vi "Hall of Bar sample Test.vi"(8 "error in (no error)":errorcluster) -> (0 "error out":errorcluster)   [LabVIEW 2016, in "Hall Effect Library.lvlib"]
uses:
  Hall Effect Library.lvlib
  Controls/Measurement.ctl
  Public/Controls/Data Items.ctl
  Public/Controls/Tests.ctl
  Global Variables/Test Settings.vi
  Global Variables/Hall Effect Data.vi
  Global Variables/Instrument Locations.vi
panel:
  out "Test Step":T1(ring)
  out "Measurement":T2
  out "Soak Until":timestamp
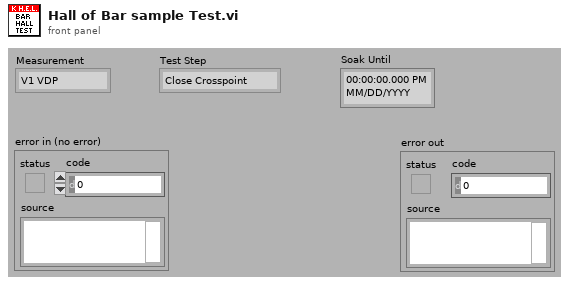
[diagram p1: front panel]
types:
  T1 = enum16{"Close Crosspoint", "Soak 1", "Zero Ammeter", "Zero Voltmeter", "I-SRC On", "Adjust potentiometer to 0V ", "Init Ammeter", "Soak 2", "Measure I", "Measure V", "I-SRC Off", "Open Crosspoint", "Done"}
  T2 = typedef "Hall Effect Library.lvlib/Measurement.ctl" = enum16{"V1 VDP", "V2 VDP", "V3 VDP", "V4 VDP", "V5 VDP", "V6 VDP", "V7 VDP", "V8 VDP", "V1 HE", "V2 HE", "V3 HE", "V4 HE", "V5 HE", "V6 HE", "V7 HE", "V8 HE", "V1 Res Bar", "V1 Hall Bar", "V1 Res 6-Cot", "V2 Res 6-Cot", "V3 Res 6-Cot", "V4 Res 6-Cot", "V1 Hall 6-Cot", "V2 Hall 6-Cot", "V3 Hall 6-Cot", "V4 Hall 6-Cot", "V5 Hall 6-Cot", "V6 Hall 6-Cot", "V7 Hall 6-Cot", "V8 Hall 6-Cot", "V1 Res 8-Cot", "V2 Res 8-Cot", "V3 Res 8-Cot", "V4 Res 8-Cot", "V1 Hall 8-Cot", "V2 Hall 8-Cot", "V3 Hall 8-Cot", "V4 Hall 8-Cot"}
  T3 = typedef "Hall Effect Library.lvlib/Resisitivity.ctl" = enum16{"Low", "High"}
  T4 = enum16{"Close Crosspoint", "Soak 1", "Zero Ammeter", "Zero Voltmeter", "I-SRC On", "Init Ammeter", "Soak 2", "Measure I", "Measure V", "I-SRC Off", "Open Crosspoint", "Done"}
  T5 = typedef "Hall Effect Library.lvlib/Tests.ctl" = enum16{"Van Der Pauw", "Hall Effect", "Bar Sample Resistivity", "Bar Sample Hall ", "6-Contact Sample Resistivity", "6-Contact Sample Hall", "8-Contact Sample Resistivity", "8-Contact Sample Hall", ""}
  T6 = typedef "Hall Effect Library.lvlib/Data Items.ctl" = enum16{"V1 Van Der Pauw", "V2 Van Der Pauw", "V3 Van Der Pauw", "V4 Van Der Pauw", "V5 Van Der Pauw", "V6 Van Der Pauw", "V7 Van Der Pauw", "V8 Van Der Pauw", "V1 Hall Effect", "V2 Hall Effect", "V3 Hall Effect", "V4 Hall Effect", "V5 Hall Effect", "V6  Hall Effect", "V7 Hall Effect", "V8 Hall Effect", "V1 Res Bar", "V1 Hall Bar", "V1 Res 6-Cot", "V2 Res 6-Cot", "V3 Res 6-Cot", "V4 Res 6-Cot", "V1 Hall 6-Cot", "V2 Hall 6-Cot", "V3 Hall 6-Cot", "V4 Hall 6-Cot", "V5 Hall 6-Cot", "V6 Hall 6-Cot", "V7 Hall 6-Cot", "V8 Hall 6-Cot", "V1 Res 8-Cot", "V2 Res 8-Cot", "V3 Res 8-Cot", "V4 Res 8-Cot", "V1 Hall 8-Cot", "V2 Hall 8-Cot", "V3 Hall 8-Cot", "V4 Hall 8-Cot", "Van Der Pauw Results", "Hall Effect Results", "Bar Sample Resistivity Results", "Bar Sample Hall Results", "6-Contact Resistivity Results", "6-Contact Hall Results", "8-Contact Resistivity Results", "8-Contact Hall Results"}
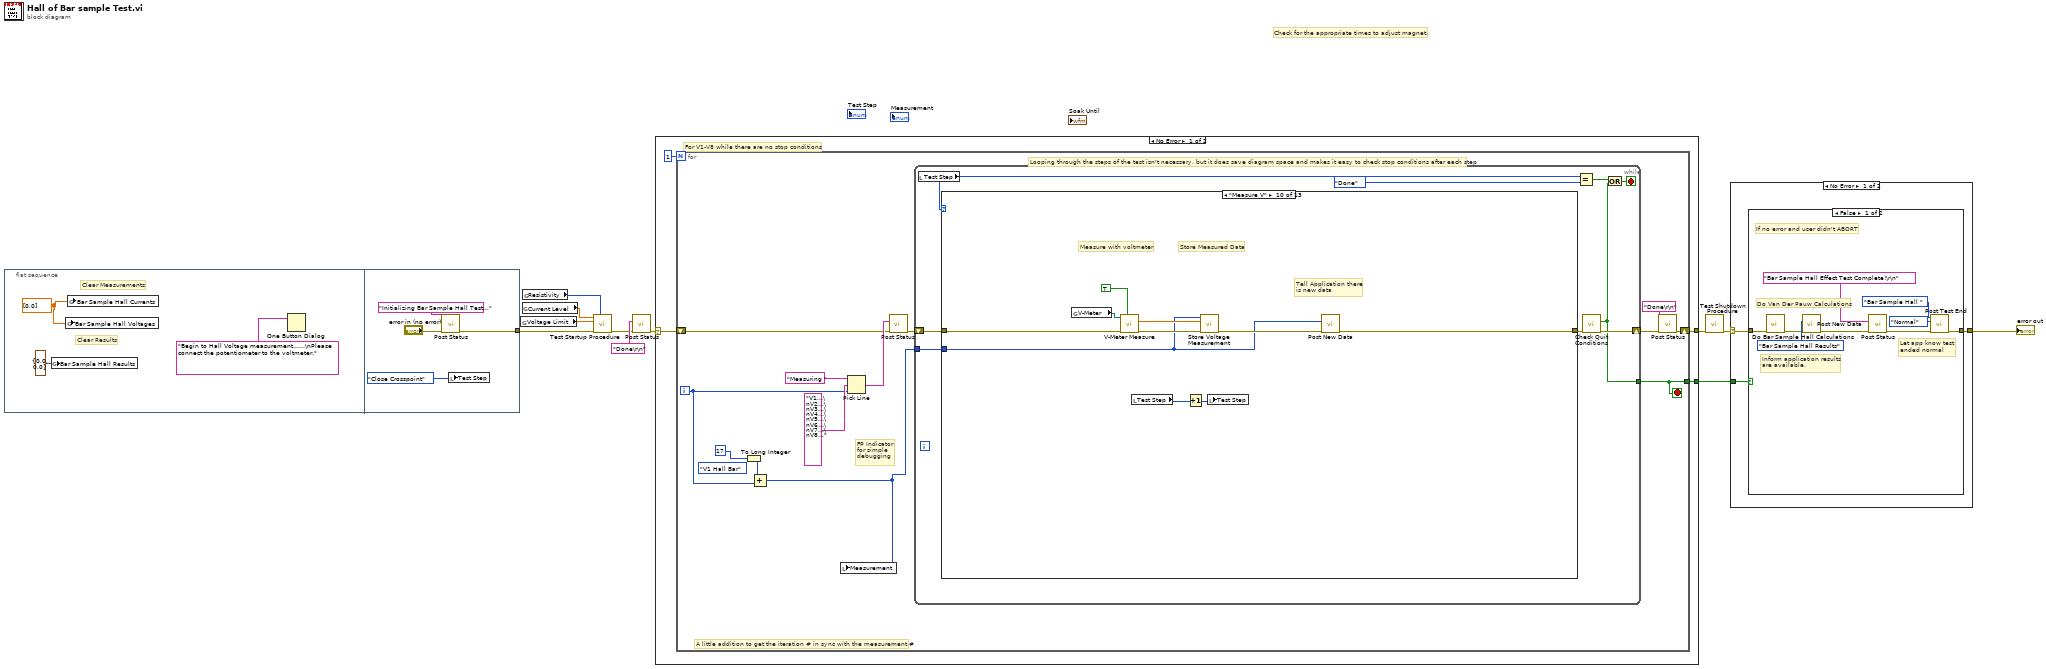
[diagram p0: block diagram]
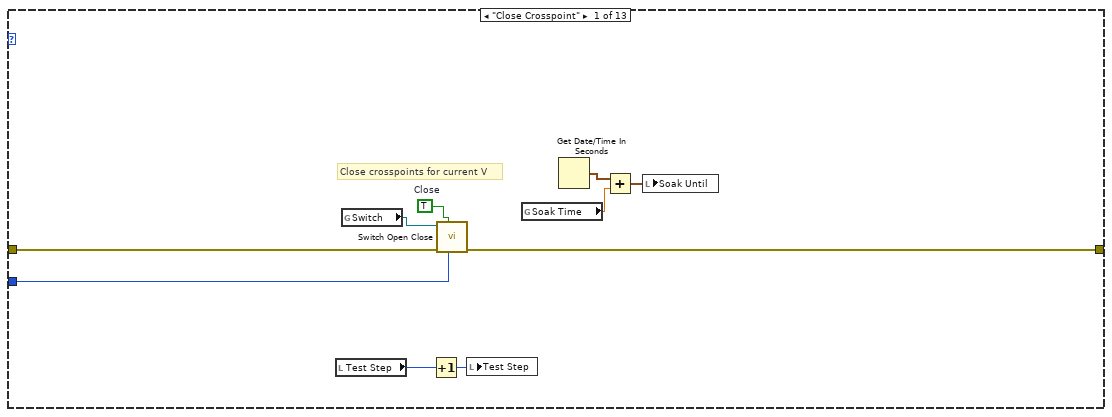
[diagram p2: hidden frame]
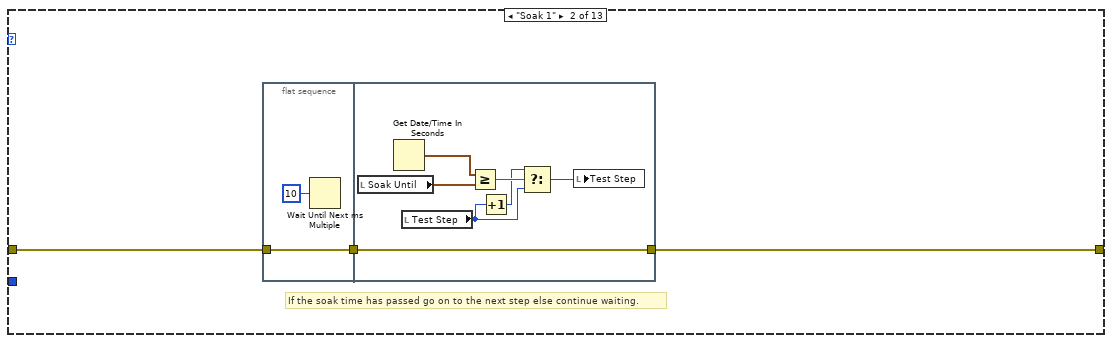
[diagram p3: hidden frame]
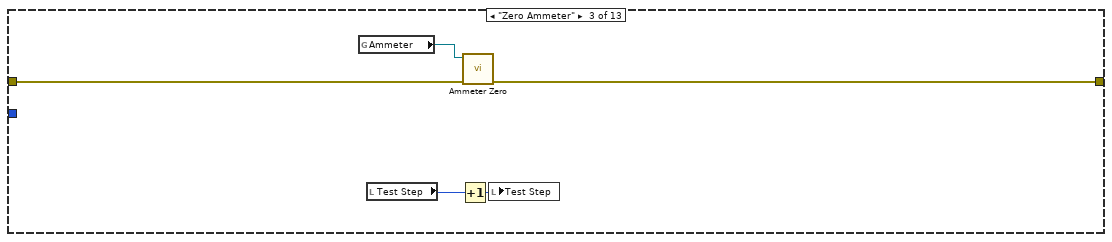
[diagram p4: hidden frame]
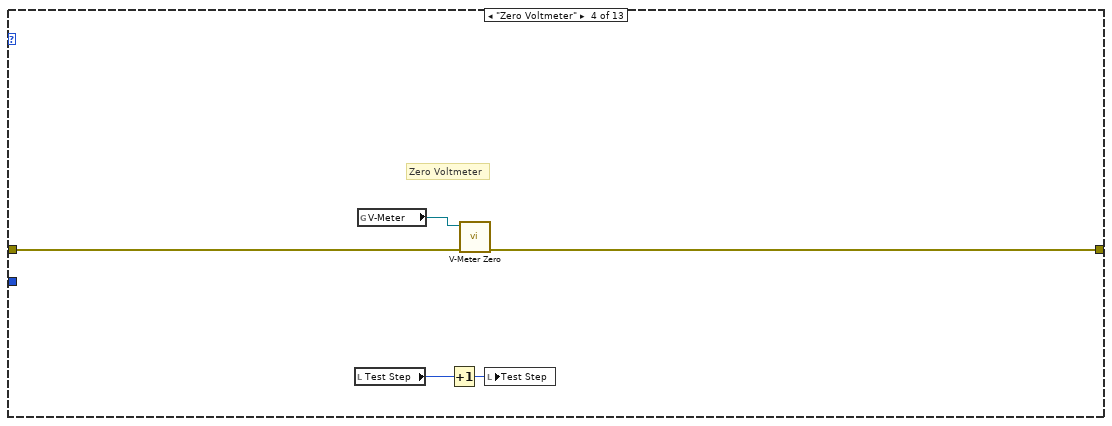
[diagram p5: hidden frame]
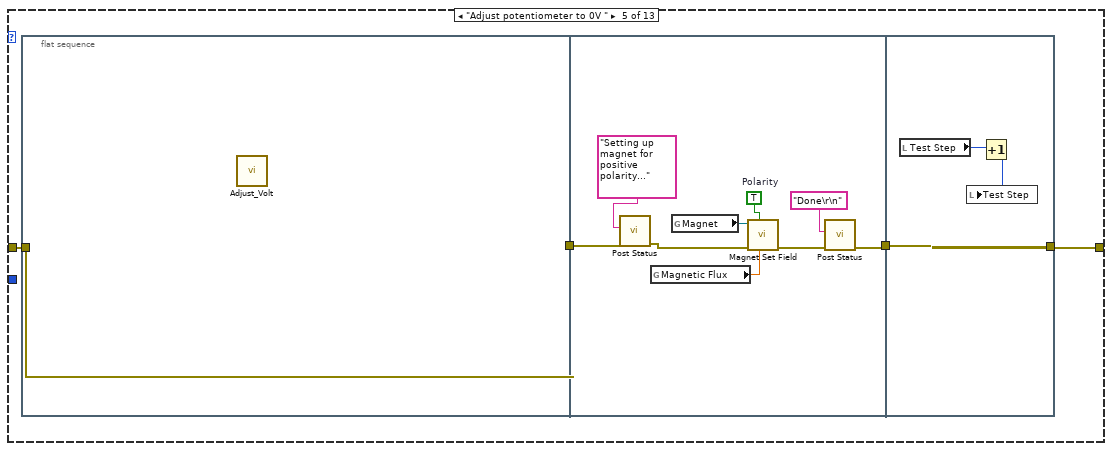
[diagram p6: hidden frame]
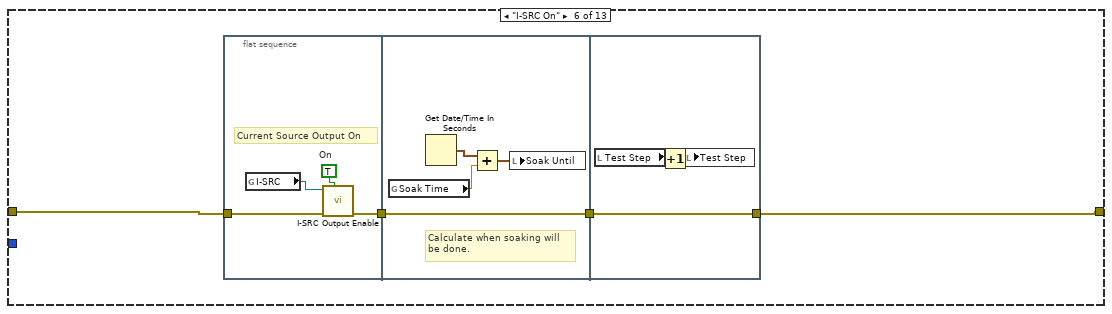
[diagram p7: hidden frame]
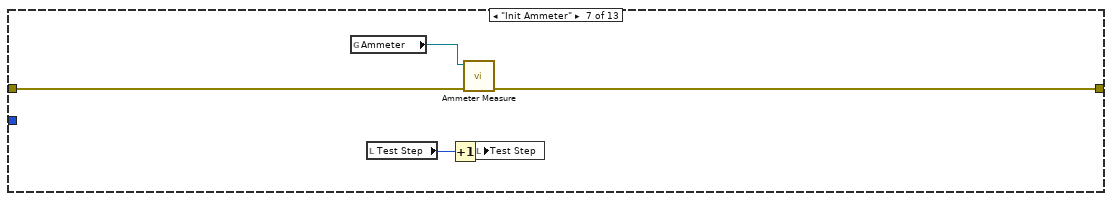
[diagram p8: hidden frame]
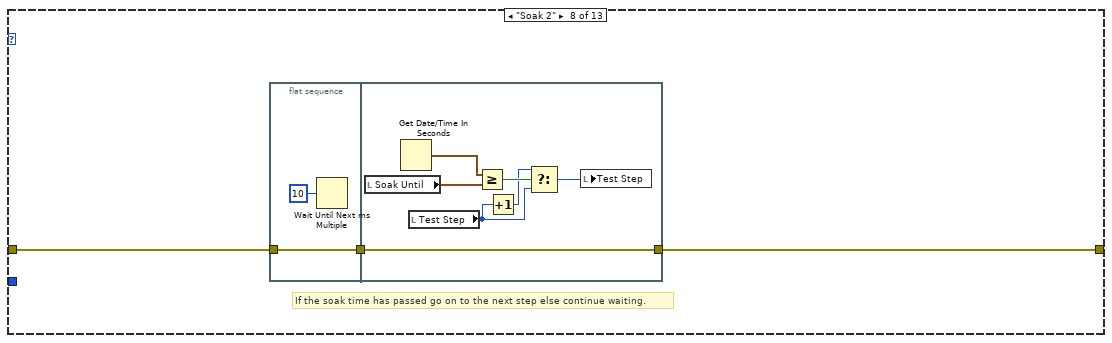
[diagram p9: hidden frame]
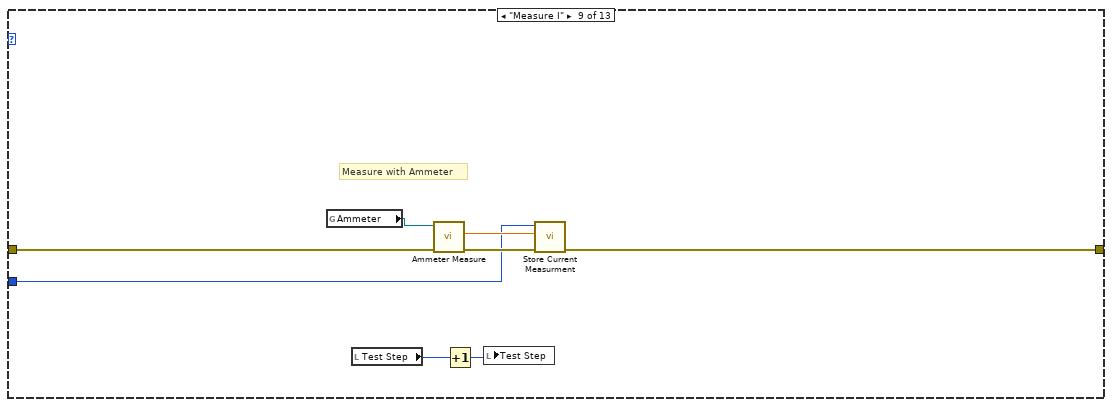
[diagram p10: hidden frame]
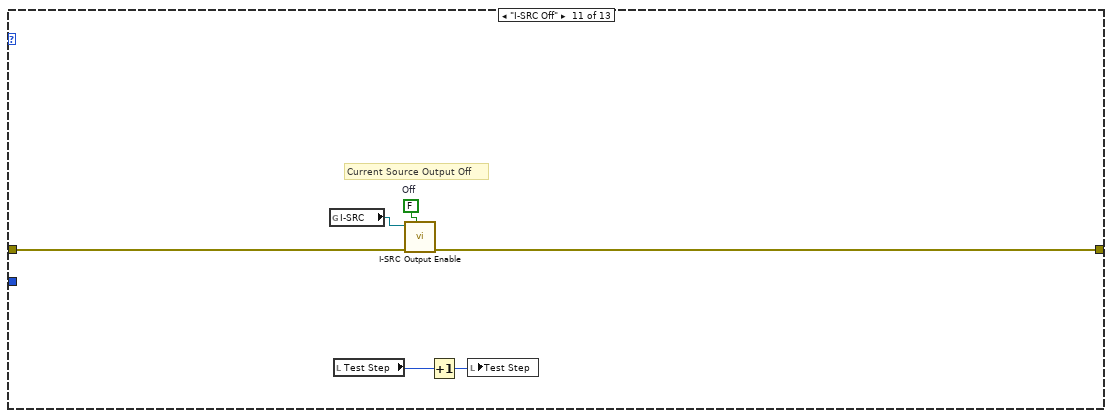
[diagram p11: hidden frame]
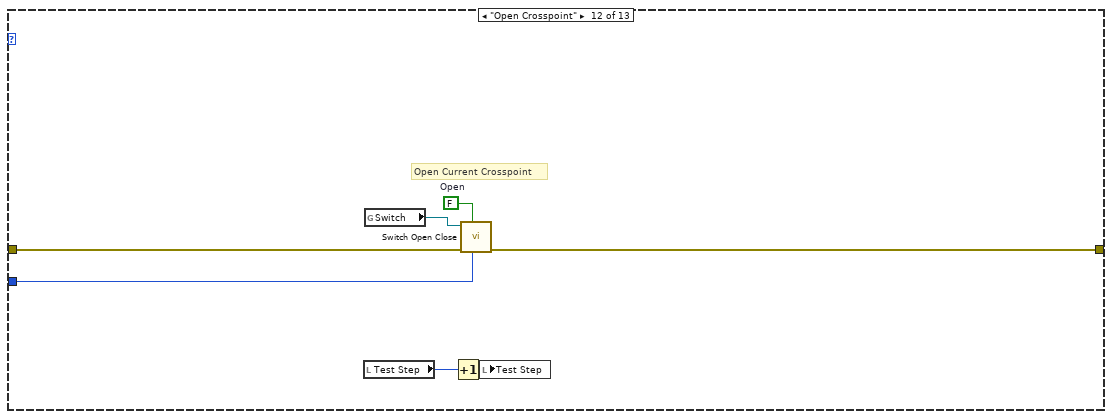
[diagram p12: hidden frame]
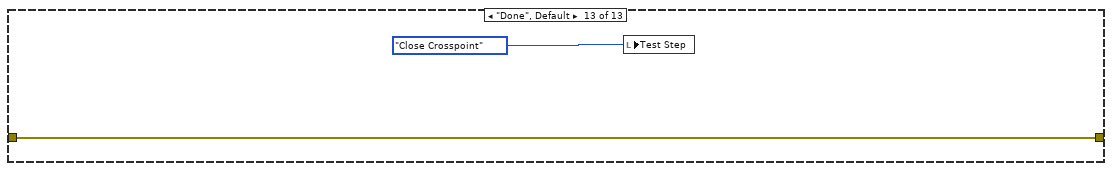
[diagram p13: hidden frame]
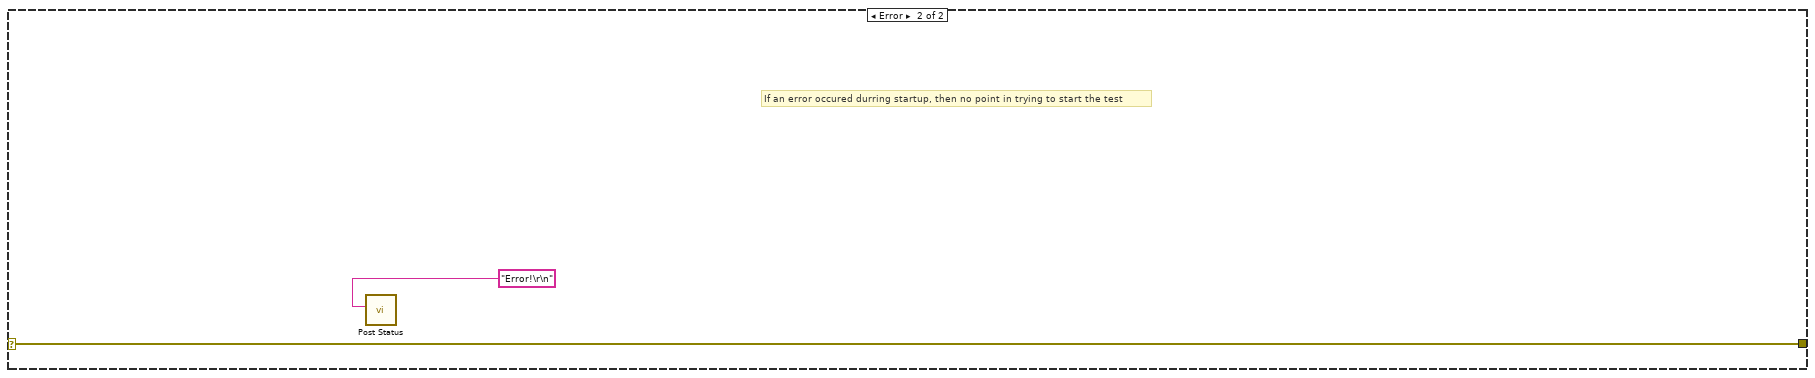
[diagram p14: hidden frame]
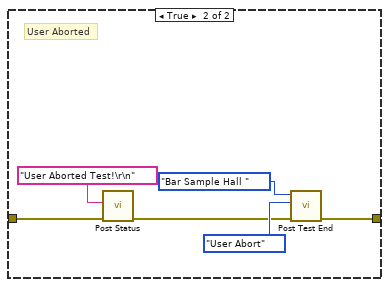
[diagram p15: hidden frame]
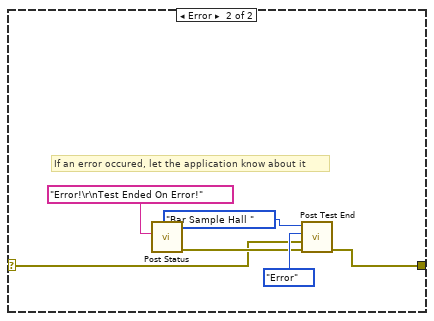
[diagram p16: hidden frame]
diagram:
  # "Check for the appropriate times to adjust magnet."
  n1 = flat-sequence {
    tunnel: [w18] -> w5
    frame #0 {
      w14 = dbl[] [0.0] ("Bar Sample Hall Currents")
      # "Clear Results"
      # "Clear Measurements"
      n2 = global write "Hall Effect Data.vi" "Bar Sample Hall Results"(cluster{"n/p":dbl, "uH":dbl} {"n/p"=0.0, "uH"=0.0} ("Bar Sample Hall Results")) -> ()
      n3 = global write "Hall Effect Data.vi" "Bar Sample Hall Voltages"(w14) -> ()
      n4 = global write "Hall Effect Data.vi" "Bar Sample Hall Currents"(w14) -> ()
      n5 = One Button Dialog(message="Begin to Hall Voltage measurement......\nPlease connect the potentiometer to the voltmeter.") -> ()  [unwired: 1 in, 1 out]
    }
    frame #1 {
      n6 = call "Post Status.vi"("error in (no error)"="error in (no error)", "Status Message"="Initializing Bar Sample Hall Test...") -> ("error out"=w18:errorcluster)  [unwired: 9 out]
      n7 = local write "Test Step"(T1."Close Crosspoint" ("Test Step")) -> ()
    }
  }
  n8 = global read "Test Settings.vi" "Voltage Limit"() -> (w6:dbl)
  n9 = global read "Test Settings.vi" "Current Level"() -> (w7:dbl)
  n10 = global read "Test Settings.vi" "Resistivity"() -> (w8:T3)
  n11 = call "Test Startup Procedure.vi"("Resistivity"=w8, "error in (no error)"=w5, "Voltage Limit"=w6, "Current Level"=w7) -> ("error out"=w3:errorcluster)  [unwired: 7 out]
  n12 = call "Post Status.vi"("error in (no error)"=w3, "Status Message"="Done\r\n") -> ("error out"=w9:errorcluster)  [unwired: 9 out]
  n13 = case shown="No Error" w9 {
    selector: w9 -> [w20 w160]
    tunnel: [w22 w160] -> w2
    tunnel: [w21 _] -> w10
    frame No Error {
      # "For V1-V8 while there are no stop conditions"
      n14 = for {
        N: 1 -> [_]
        shift-right: [w28] -> w22
        shift-left: w20 -> [w24]
        tunnel: [w25] -> w21
        i -> [w30]
        stop <- w25 stop-if-true
        (unwired) Measurement."V1 Hall Bar" ("Measurement")
        # "A little addition to get the iteration # in sync with the measurement #"
        # "FP Indicator\nfor simple\ndebugging"
        # "Looping through the steps of the test isn't necessary, but it does save diagram space and makes it easy to check stop conditions after each step"
        n15 = To Long Integer(number=17) -> (32bit integer=w31:i32)
        n16 = Add(x=w31, y=w30) -> (x+y=w26:i32)
        n17 = local write "Measurement"(w26) -> ()
        n18 = Pick Line(string ("")="Measuring ", multi-line string="V1...\nV2...\nV3...\nV4...\nV5...\nV6...\nV7...\nV8...", line index=w30) -> (output string=w33:string)
        n19 = call "Post Status.vi"("error in (no error)"=w24, "Status Message"=w33) -> ("error out"=w32:errorcluster)  [unwired: 9 out]
        n20 = while {
          shift-right: [w42] -> w27
          shift-left: w32 -> [w44]
          tunnel: w26 -> [w43]
          tunnel: [w38] -> w25
          stop <- w41 stop-if-true
          n21 = local read "Test Step"() -> (w39:T1)
          n22 = case shown="\"Measure V\"" w39 {
            tunnel: [w52 w55 w70 w74 w79 w96 w112 w115 w130 w138 w146 w154 w158] -> w37
            tunnel: w44 -> [w51 w56 w71 w75 w80 w97 w113 w116 w132 w142 w147 w153 w158]
            tunnel: w43 -> [w50 _ _ _ _ _ _ _ w128 w137 _ w152 _]
            frame "Close Crosspoint" {
              w53 = TRUE  # Close
              # "Close crosspoints for current V"
              n23 = local read "Test Step"() -> (w48:T1)
              n24 = global read "Instrument Locations.vi" "Switch"() -> (w54:refnum<visa-resource-name>)
              n25 = Increment(x=w48) -> (x+1=w49:T1)
              n26 = call "Switch Open Close.vi"("Measurement"=w50, "Open/Close (F: Open)"=w53, "error in (no error)"=w51, "VISA resource name in"=w54) -> ("error out"=w52:errorcluster)  [unwired: 7 out]
              n27 = local write "Test Step"(w49) -> ()
              n28 = global read "Test Settings.vi" "Soak Time"() -> (w46:dbl)
              n29 = Get Date/Time In Seconds() -> (seconds since 1Jan1904=w45:timestamp)
              n30 = Add(x=w45, y=w46) -> (x+y=w47:timestamp)
              n31 = local write "Soak Until"(w47) -> ()
            }
            frame "Soak 1" {
              # "If the soak time has passed go on to the next step else continue waiting."
              n32 = flat-sequence {
                tunnel: w56 -> [w58]
                tunnel: [w58] -> w57
                tunnel: [w62] -> w55
                tunnel: w57 -> [w62]
                frame #0 {
                  n33 = Wait Until Next ms Multiple(millisecond multiple=u32 10) -> ()  [unwired: 1 out]
                }
                frame #1 {
                  n34 = local read "Soak Until"() -> (w65:timestamp)
                  n35 = Get Date/Time In Seconds() -> (seconds since 1Jan1904=w66:timestamp)
                  n36 = local read "Test Step"() -> (w60:T1)
                  n37 = Greater Or Equal?(x=w66, y=w65) -> (x >= y?=w64:bool)
                  n38 = Increment(x=w60) -> (x+1=w61:T1)
                  n39 = Select(t=w61, s=w64, f=w60) -> (s? t:f=w63:T1)
                  n40 = local write "Test Step"(w63) -> ()
                }
              }
            }
            frame "Zero Ammeter" {
              n41 = global read "Instrument Locations.vi" "Ammeter"() -> (w69:refnum<visa-resource-name>)
              n42 = local read "Test Step"() -> (w67:T1)
              n43 = Increment(x=w67) -> (x+1=w68:T1)
              n44 = call "Ammeter Zero.vi"("error in (no error)"=w71, "VISA resource name in"=w69) -> ("error out"=w70:errorcluster)  [unwired: 9 out]
              n45 = local write "Test Step"(w68) -> ()
            }
            frame "Zero Voltmeter" {
              # "Zero Voltmeter"
              n46 = local read "Test Step"() -> (w73:T1)
              n47 = global read "Instrument Locations.vi" "V-Meter"() -> (w76:refnum<visa-resource-name>)
              n48 = Increment(x=w73) -> (x+1=w72:T1)
              n49 = call "V-Meter Zero.vi"("error in (no error)"=w75, "VISA resource name in"=w76) -> ("error out"=w74:errorcluster)  [unwired: 9 out]
              n50 = local write "Test Step"(w72) -> ()
            }
            frame "Adjust potentiometer to 0V " {
              n51 = flat-sequence {
                tunnel: w80 -> [w81]
                tunnel: [w81] -> w78
                tunnel: w78 -> [w83]
                tunnel: [w82] -> w77
                tunnel: w77 -> [w91]
                tunnel: [w91] -> w79
                frame #0 {
                  n52 = call "Adjust_Volt.vi"() -> ()  [unwired: 12 in]
                }
                frame #1 {
                  w88 = TRUE  # Polarity
                  n53 = call "Post Status.vi"("error in (no error)"=w83, "Status Message"="Setting up magnet for positive polarity...") -> ("error out"=w85:errorcluster)  [unwired: 9 out]
                  n54 = global read "Test Settings.vi" "Magnetic Flux"() -> (w86:dbl)
                  n55 = global read "Instrument Locations.vi" "Magnet"() -> (w87:refnum<visa-resource-name>)
                  n56 = call "Magnet Set Field.vi"("Field Strength"=w86, "Polarity"=w88, "error in (no error)"=w85, "VISA resource name in"=w87) -> ("error out"=w84:errorcluster)  [unwired: 7 out]
                  n57 = call "Post Status.vi"("error in (no error)"=w84, "Status Message"="Done\r\n") -> ("error out"=w82:errorcluster)  [unwired: 9 out]
                }
                frame #2 {
                  n58 = local read "Test Step"() -> (w93:T1)
                  n59 = Increment(x=w93) -> (x+1=w92:T1)
                  n60 = local write "Test Step"(w92) -> ()
                }
              }
            }
            frame "I-SRC On" {
              n61 = flat-sequence {
                tunnel: [w98] -> w95
                tunnel: w97 -> [w99]
                tunnel: w95 -> [w105]
                tunnel: [w105] -> w94
                tunnel: [w108] -> w96
                tunnel: w94 -> [w108]
                frame #0 {
                  w100 = TRUE  # On
                  # "Current Source Output On"
                  n62 = global read "Instrument Locations.vi" "I-SRC"() -> (w101:refnum<visa-resource-name>)
                  n63 = call "I-SRC Output Enable.vi"("Output (Off)"=w100, "error in (no error)"=w99, "VISA resource name in"=w101) -> ("error out"=w98:errorcluster)  [unwired: 8 out]
                }
                frame #1 {
                  # "Calculate when soaking will\nbe done."
                  n64 = global read "Test Settings.vi" "Soak Time"() -> (w103:dbl)
                  n65 = Get Date/Time In Seconds() -> (seconds since 1Jan1904=w102:timestamp)
                  n66 = Add(x=w102, y=w103) -> (x+y=w104:timestamp)
                  n67 = local write "Soak Until"(w104) -> ()
                }
                frame #2 {
                  n68 = local read "Test Step"() -> (w107:T1)
                  n69 = Increment(x=w107) -> (x+1=w106:T1)
                  n70 = local write "Test Step"(w106) -> ()
                }
              }
            }
            frame "Init Ammeter" {
              n71 = global read "Instrument Locations.vi" "Ammeter"() -> (w111:refnum<visa-resource-name>)
              n72 = local read "Test Step"() -> (w110:T1)
              n73 = Increment(x=w110) -> (x+1=w109:T1)
              n74 = call "Ammeter Measure.vi"("error in (no error)"=w113, "VISA resource name in"=w111) -> ("error out"=w112:errorcluster)  [unwired: 9 out]
              n75 = local write "Test Step"(w109) -> ()
            }
            frame "Soak 2" {
              # "If the soak time has passed go on to the next step else continue waiting."
              n76 = flat-sequence {
                tunnel: w116 -> [w117]
                tunnel: [w117] -> w114
                tunnel: [w121] -> w115
                tunnel: w114 -> [w121]
                frame #0 {
                  n77 = Wait Until Next ms Multiple(millisecond multiple=u32 10) -> ()  [unwired: 1 out]
                }
                frame #1 {
                  n78 = local read "Soak Until"() -> (w124:timestamp)
                  n79 = Get Date/Time In Seconds() -> (seconds since 1Jan1904=w125:timestamp)
                  n80 = local read "Test Step"() -> (w119:T1)
                  n81 = Greater Or Equal?(x=w125, y=w124) -> (x >= y?=w123:bool)
                  n82 = Increment(x=w119) -> (x+1=w120:T1)
                  n83 = Select(t=w120, s=w123, f=w119) -> (s? t:f=w122:T1)
                  n84 = local write "Test Step"(w122) -> ()
                }
              }
            }
            frame "Measure I" {
              # "Measure with Ammeter"
              n85 = global read "Instrument Locations.vi" "Ammeter"() -> (w133:refnum<visa-resource-name>)
              n86 = local read "Test Step"() -> (w127:T1)
              n87 = call "Ammeter Measure.vi"("error in (no error)"=w132, "VISA resource name in"=w133) -> ("error out"=w131:errorcluster, "Measurement"=w129:dbl)  [unwired: 8 out]
              n88 = Increment(x=w127) -> (x+1=w126:T1)
              n89 = local write "Test Step"(w126) -> ()
              n90 = call "Store Current Measurment.vi"("error in"=w131, "Value"=w129, "Measurement"=w128) -> ("error out"=w130:errorcluster)  [unwired: 8 out]
            }
            frame "Measure V" {
              # "Tell Application there\nis new data"
              # "Store Measured Data"
              # "Measure with voltmeter"
              n91 = global read "Instrument Locations.vi" "V-Meter"() -> (w143:refnum<visa-resource-name>)
              n92 = call "V-Meter Measure.vi"("Boolean"=TRUE, "error in (no error)"=w142, "VISA resource name in"=w143) -> ("error out"=w141:errorcluster, "Measurement"=w140:dbl)  [unwired: 7 out]
              n93 = local read "Test Step"() -> (w135:T1)
              n94 = Increment(x=w135) -> (x+1=w136:T1)
              n95 = call "Store Voltage Measurement.vi"("error in"=w141, "Value"=w140, "Measurement"=w137) -> ("error out"=w139:errorcluster)  [unwired: 8 out]
              n96 = local write "Test Step"(w136) -> ()
              n97 = call "Post New Data.vi"("error in (no error)"=w139, "Data Item"=w137) -> ("error out"=w138:errorcluster)  [unwired: 9 out]
            }
            frame "I-SRC Off" {
              w148 = FALSE  # Off
              # "Current Source Output Off"
              n98 = global read "Instrument Locations.vi" "I-SRC"() -> (w149:refnum<visa-resource-name>)
              n99 = local read "Test Step"() -> (w145:T1)
              n100 = call "I-SRC Output Enable.vi"("Output (Off)"=w148, "error in (no error)"=w147, "VISA resource name in"=w149) -> ("error out"=w146:errorcluster)  [unwired: 8 out]
              n101 = Increment(x=w145) -> (x+1=w144:T1)
              n102 = local write "Test Step"(w144) -> ()
            }
            frame "Open Crosspoint" {
              w155 = FALSE  # Open
              # "Open Current Crosspoint"
              n103 = local read "Test Step"() -> (w151:T1)
              n104 = global read "Instrument Locations.vi" "Switch"() -> (w156:refnum<visa-resource-name>)
              n105 = Increment(x=w151) -> (x+1=w150:T1)
              n106 = call "Switch Open Close.vi"("Measurement"=w152, "Open/Close (F: Open)"=w155, "error in (no error)"=w153, "VISA resource name in"=w156) -> ("error out"=w154:errorcluster)  [unwired: 7 out]
              n107 = local write "Test Step"(w150) -> ()
            }
            frame "Done", Default {
              n108 = local write "Test Step"(T1."Close Crosspoint" ("Test Step")) -> ()
            }
          }
          n109 = Equal?(x=w39, y=T4."Done") -> (x = y?=w40:bool)
          n110 = call "Check Quit Conditions.vi"("error in (no error)"=w37) -> ("error out"=w42:errorcluster, "Quit?"=w38:bool)  [unwired: 9 out]
          n111 = Or(x=w40, y=w38) -> (x .or. y?=w41:bool)
        }
        n112 = call "Post Status.vi"("error in (no error)"=w27, "Status Message"="Done\r\n") -> ("error out"=w28:errorcluster)  [unwired: 9 out]
      }
    }
    frame Error {
      # "If an error occured durring startup, then no point in trying to start the test"
      n113 = call "Post Status.vi"("Status Message"="Error!\r\n") -> ()  [unwired: 1 in, 10 out]
    }
  }
  n114 = call "Test Shutdown Procedure.vi"("error in (no error)"=w2) -> ("error out"=w1:errorcluster)  [unwired: 10 out]
  n115 = case shown="No Error" w1 {
    selector: w1 -> [w162 w180]
    tunnel: w10 -> [w163 _]
    tunnel: [w161 w181] -> w11
    frame No Error {
      n116 = case shown="False" w163 {
        tunnel: w162 -> [w165 w177]
        tunnel: [w167 w174] -> w161
        frame False {
          # "Let app know test\nended normal"
          # "Inform application results\nare available."
          # "Do Van Der Pauw Calculations"
          # "If no error and user didn't ABORT"
          n117 = call "Do Bar Sample Hall Calculations.vi"("error in (no error)"=w165) -> ("error out"=w164:errorcluster)  [unwired: 10 in]
          n118 = call "Post New Data.vi"("error in (no error)"=w164, "Data Item"=Data_Items."Bar Sample Hall Results") -> ("error out"=w170:errorcluster)  [unwired: 9 out]
          n119 = call "Post Status.vi"("error in (no error)"=w170, "Status Message"="Bar Sample Hall Effect Test Complete!\r\n") -> ("error out"=w169:errorcluster)  [unwired: 9 out]
          n120 = call "Post Test End.vi"("error in (no error)"=w169, "Test End"=enum16{"Normal", "User Abort", "Error"}."Normal", "Test"=Tests."Bar Sample Hall ") -> ("error out"=w167:errorcluster)  [unwired: 1 in, 7 out]
        }
        frame True {
          # "User Aborted"
          n121 = call "Post Status.vi"("error in (no error)"=w177, "Status Message"="User Aborted Test!\r\n") -> ("error out"=w176:errorcluster)  [unwired: 9 out]
          n122 = call "Post Test End.vi"("error in (no error)"=w176, "Test End"=enum16{"Normal", "User Abort", "Error"}."User Abort", "Test"=Tests."Bar Sample Hall ") -> ("error out"=w174:errorcluster)  [unwired: 1 in, 7 out]
        }
      }
    }
    frame Error {
      # "If an error occured, let the application know about it"
      n123 = call "Post Status.vi"("Status Message"="Error!\r\nTest Ended On Error!") -> ("error out"=w183:errorcluster)  [unwired: 1 in, 9 out]
      n124 = call "Post Test End.vi"("error in (no error)"=w183, "Test End Error (no error)"=w180, "Test End"=enum16{"Normal", "User Abort", "Error"}."Error", "Test"=Tests."Bar Sample Hall ") -> ("error out"=w181:errorcluster)  [unwired: 7 out]
    }
  }
  "error out" <- w11
